vi "Move axes to their middle position.vi"(0 "System no.":i32=1 min=1 max=4 step=1, 1 "All axes?":bool, 2 "Axes to command":string[](array[string]), 5 "error in":errorcluster, 12 "Stop refnum":refnum<vi>) -> (14 "Position":dbl[](array[numeric]) format="%.6f", 19 "error out":errorcluster)   [LabVIEW 2020]
doc: "Moves axes to the middle position of their travel range, waits until motion has finished and queries position. VI also stops if Stop refnum or Local stop is TRUE. When using as a sub-VI, use Stop refnum to stop VI from caller."
panel:
  in  "stop":bool
  # "Moves axes to the middle position of their travel range."
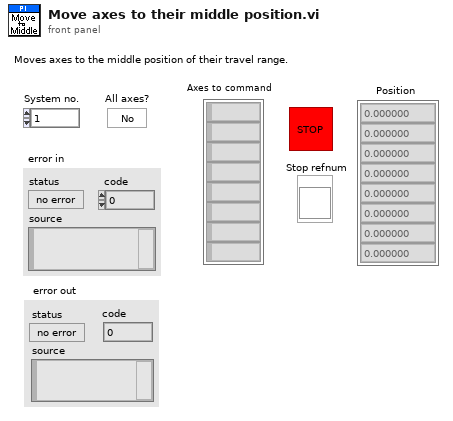
[diagram p1: front panel]
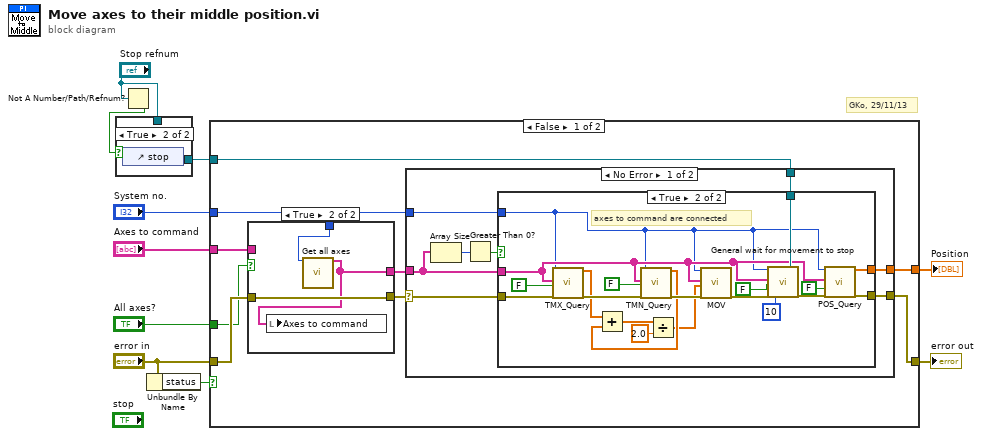
[diagram p0: block diagram]
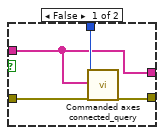
[diagram p3: hidden frame]
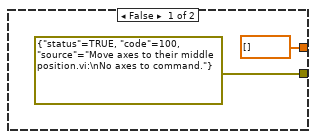
[diagram p4: hidden frame]
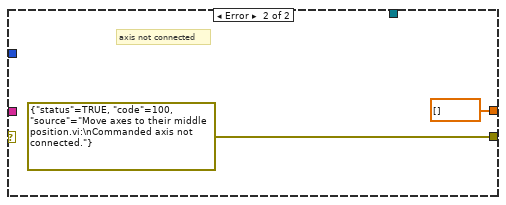
[diagram p5: hidden frame]
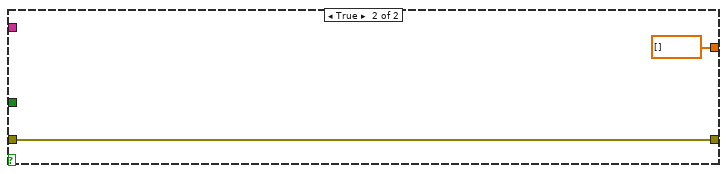
[diagram p6: hidden frame]
diagram:
  # "GKo, 29/11/13"
  n1 = Not A Number/Path/Refnum?(number/path/refnum="Stop refnum") -> (NaN/Path/Refnum?=w4:bool)
  n2 = case shown="True" w4 {
    tunnel: [w11 w12] -> w2
    tunnel: "Stop refnum" -> [w11 _]
    frame False {
    }
    frame True {
      n3 = control-ref of="stop"() -> (w12:refnum<vi>)
    }
  }
  n4 = Unbundle By Name("error in") -> ("status"=w6:bool)
  n5 = case shown="False" w6 {
    tunnel: [w21 w62] -> w10
    tunnel: "error in" -> [w20 w62]
    tunnel: "System no." -> [w17 _]
    tunnel: "Axes to command" -> [w19 _]
    tunnel: "All axes?" -> [w18 _]
    tunnel: w2 -> [w14 _]
    tunnel: [w13 dbl[] [] ("Position")] -> w1
    frame False {
      n6 = case shown="True" w18 {
        tunnel: [w22 w26] -> w15
        tunnel: w20 -> [w25 w27]
        tunnel: [w24 w27] -> w16
        tunnel: w17 -> [w23 w28]
        tunnel: w19 -> [w22 _]
        frame False {
          n7 = call "Commanded axes connected_query.vi"("System no."=w23, "Commanded axes"=w22, "error in"=w25) -> ("error out"=w24:errorcluster)  [unwired: 1 in, 15 out]
        }
        frame True {
          n8 = call "Get all axes.vi"("System no."=w28) -> ("Conn. Axes"=w26:string[])  [unwired: 18 out]
          n9 = local write "Axes to command"(w26) -> ()
        }
      }
      n10 = case shown="No Error" w16 {
        selector: w16 -> [w34 _]
        tunnel: w15 -> [w32 _]
        tunnel: [w30 errorcluster {"status"=TRUE, "code"=100, "source"="Move axes to their middle position.vi:\nCommanded axis not connected."} ("error out")] -> w21
        tunnel: w17 -> [w33 _]
        tunnel: w14 -> [w31 _]
        tunnel: [w29 dbl[] [] ("Position")] -> w13
        frame No Error {
          n11 = Array Size(array=w32) -> (size(s)=w36:i32)
          n12 = Greater Than 0?(x=w36) -> (x > 0?=w35:bool)
          n13 = case shown="True" w35 {
            tunnel: w34 -> [_ w58]
            tunnel: w33 -> [_ w46]
            tunnel: w32 -> [_ w47]
            tunnel: w31 -> [_ w49]
            tunnel: [errorcluster {"status"=TRUE, "code"=100, "source"="Move axes to their middle position.vi:\nNo axes to command."} ("error out") w44] -> w30
            tunnel: [dbl[] [] ("Position") w43] -> w29
            frame False {
            }
            frame True {
              # "axes to command are connected"
              n14 = call "TMX_Query.vi"("System no."=w46, "Axes to query"=w47, "All axes?"=FALSE, "error in"=w58) -> ("Maximum travel limit"=w53:dbl[], "error out"=w56:errorcluster)  [unwired: 1 in, 13 out]
              n15 = call "TMN_Query.vi"("System no."=w46, "Axes to query"=w47, "All axes?"=FALSE, "error in"=w56) -> ("Minimum travel limit"=w52:dbl[], "error out"=w54:errorcluster)  [unwired: 1 in, 13 out]
              n16 = Add(x=w53, y=w52) -> (x+y=w41:dbl[])
              n17 = Divide(x=w41, y=2.0) -> (x/y=w39:dbl[])
              n18 = call "MOV.vi"("System no."=w46, "Axes to move"=w47, "Position values"=w39, "error in"=w54) -> ("error out"=w51:errorcluster)  [unwired: 1 in, 14 out]
              n19 = call "General wait for movement to stop.vi"("System no."=w46, "Axes to wait for"=w47, "All axes?"=FALSE, "error in"=w51, "Polling cycle \ntime, ms"=u32 10 ("Polling cycle \ntime, ms"), "Stop refnum"=w49) -> ("error out"=w48:errorcluster)  [unwired: 2 in, 11 out]
              n20 = call "POS_Query.vi"("System no."=w46, "Axes to query"=w47, "All axes?"=FALSE, "error in"=w48) -> ("Position"=w43:dbl[], "error out"=w44:errorcluster)  [unwired: 1 in, 13 out]
            }
          }
        }
        frame Error {
          # "axis not connected"
        }
      }
    }
    frame True {
    }
  }
  "error out" <- w10
  "Position" <- w1
